vi "myRIO_BRig_RT_dataLick_init.vi"() -> (3 "output_dataLick":u16[][](array[numeric]))   [LabVIEW 2014]
panel:
  # "0 - iBlock\n1 - iTrial\n2 - Left (1) / Right (2) / Both (3)\n3 - iState at lick\n4 - iState after lick\n5 - Time after lick"
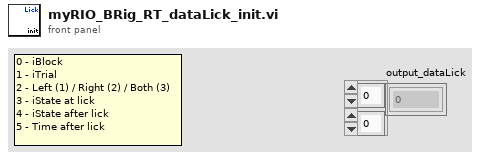
[diagram p1: front panel]
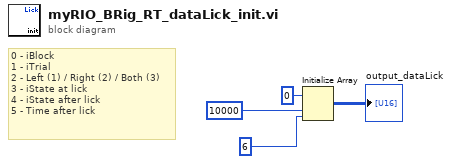
[diagram p0: block diagram]
diagram:
  # "0 - iBlock\n1 - iTrial\n2 - Left (1) / Right (2) / Both (3)\n3 - iState at lick\n4 - iState after lick\n5 - Time after lick"
  n1 = Initialize Array(u16 0 ("element"), 10000 ("dimension size"), 6 ("dimension size")) -> (→"output_dataLick":u16[][])
